vi "Actual Pressure.vi"(8 "Error In":errorcluster, 11 "VISA resource name":refnum<visa-resource-name>) -> (0 "Error Out":errorcluster, 1 "Actual Pressure":dbl, 3 "dup VISA resource name":refnum<visa-resource-name>)   [LabVIEW 2011, in "MGC647C.lvlib"]
doc: "Read actual pressure."
uses:
  <instrlib>/MGC647C/MGC647C.lvlib
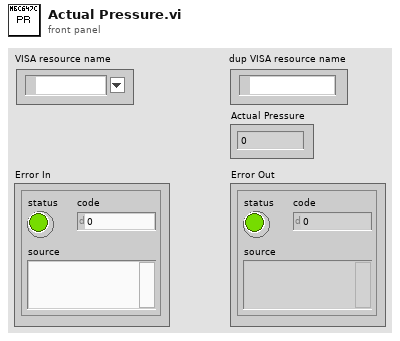
[diagram p1: front panel]
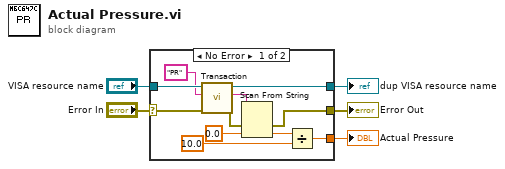
[diagram p0: block diagram]
diagram:
  n1 = case shown="No Error" "Error In" {
    selector: "Error In" -> [w7 w18]
    tunnel: "VISA resource name" -> [w16 w17]
    tunnel: [w15 w17] -> w4
    tunnel: [w14 w18] -> w3
    tunnel: [w13 _] -> w1
    frame No Error {
      n2 = call <instrlib>:"Transaction.vi"("Error In"=w7, "Command"="PR" ("string (\"\")"), "VISA resource name"=w16) -> ("Error Out"=w11:errorcluster, "Response"=w12:string, "dup VISA resource name"=w15:refnum<visa-resource-name>)  [unwired: 6 in]
      n3 = Scan From String(input string=w12, error in=w11, default 1=0.0 ("default value 1")) -> (error out=w14:errorcluster, output 1=w10:dbl)  [unwired: 2 in, 2 out]
      n4 = Divide(x=w10, y=10.0) -> (x/y=w13:dbl)
    }
    frame Error {
    }
  }
  "dup VISA resource name" <- w4
  "Error Out" <- w3
  "Actual Pressure" <- w1
